vi "Browse to URL.vi"(8 "error in":errorcluster, 11 "URL":string="http://www.ni.com/china") -> (0 "error out":errorcluster)   [LabVIEW 2011]
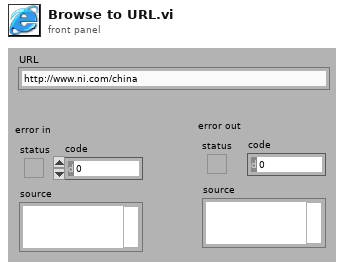
[diagram p1: front panel]
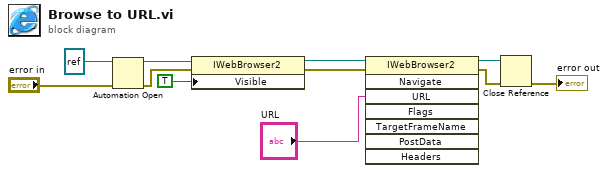
[diagram p0: block diagram]
diagram:
  n1 = Automation Open(error in (no error)="error in", Automation Refnum=refnum<k7> refnum ("SHDocVw.IWebBrowser2")) -> (Automation Refnum=w4:refnum<k7>, error out=w5:errorcluster)  [unwired: 2 in]
  n2 = property class="IWebBrowser2"(reference=w4, error in=w5, "Visible"=TRUE) -> (reference out=w7:refnum<k7>, error out=w8:errorcluster)
  n3 = invoke class="IWebBrowser2" method="Navigate"(reference=w7, error in=w8, "URL"="URL") -> (reference out=w9:refnum<k7>, error out=w10:errorcluster)  [unwired: 5 in, 6 out]
  n4 = Close Reference(reference=w9, error in (no error)=w10) -> (error out=→"error out":errorcluster)
